vi "TDMS File Status.vi"(6 "Data Path":path=path "C:/Data", 8 "erriorIn":errorcluster, 9 "prefix":string, 11 "fileRefIn":refnum<k34>) -> (0 "error out":errorcluster, 3 "tdms file out":refnum<k34>)   [LabVIEW 2014]
uses:
  File Utilities.lvlib
panel:
  in  "nFile":bool
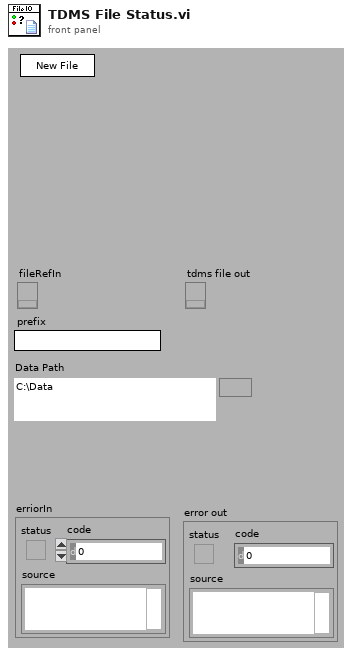
[diagram p1: front panel]
types:
  T1 = typedef "LVDateTimeRec.ctl" = cluster{"fractional second":dbl, "second":i32, "minute":i32, "hour":i32, "day of month":i32, "month":i32, "year":i32, "day of week":i32, "day of year":i32, "DST":i32}
  T2 = enum16{"open", "open or create", "create or replace", "create", "open (read-only)"}
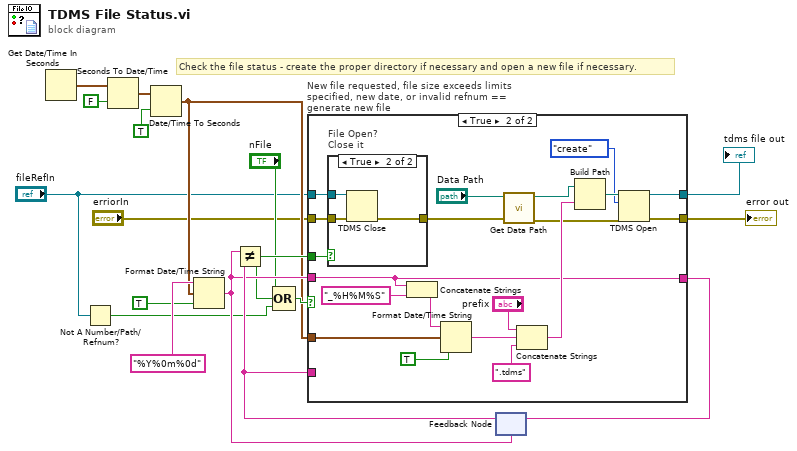
[diagram p0: block diagram]
diagram:
  # "Check the file status - create the proper directory if necessary and open a new file if necessary."
  n1 = Get Date/Time In Seconds() -> (seconds since 1Jan1904=w10:timestamp)
  n2 = Not A Number/Path/Refnum?(number/path/refnum="fileRefIn") -> (NaN/Path/Refnum?=w11:bool)
  n3 = Seconds To Date/Time(time stamp (now)=w10, to UTC (F)=FALSE) -> (date time rec=w7:T1)
  n4 = Date/Time To Seconds(1:TRUE ("is UTC (F)"), 2:w7) -> (0:w6:timestamp)
  n5 = Format Date/Time String(time format string (%c)="%Y%0m%0d", seconds (now)=w6, UTC format=TRUE) -> (date/time string=w15:string)
  n6 = feedback #1(w15) -> (w16:string)
  n7 = Not Equal?(x=w15, y=w16) -> (x != y?=w14:bool)
  n8 = Compound Arithmetic op=OR("nFile", w14, w11) -> (w13:bool)
  n9 = case "New file requested, file size exceeds limits specified, new date, or invalid refnum == generate new file" shown="True" w13 {
    tunnel: [w21 w33] -> w18
    tunnel: w15 -> [_ w33]
    tunnel: w14 -> [_ w41]
    tunnel: [w20 w24] -> w4
    tunnel: w16 -> [w21 _]
    tunnel: "erriorIn" -> [w20 w39]
    tunnel: w6 -> [_ w35]
    tunnel: [w19 w23] -> w1
    tunnel: "fileRefIn" -> [w19 w31]
    frame False {
    }
    frame True {
      n10 = case "File Open?\nClose it" shown="True" w41 {
        tunnel: [w42 w43] -> w29
        tunnel: w39 -> [w42 w45]
        tunnel: w31 -> [_ w44]
        frame False {
        }
        frame True {
          n11 = TDMS Close(8:w45, 11:w44) -> (0:w43:errorcluster)  [unwired: 1 out]
        }
      }
      n12 = Concatenate Strings(w33, "_%H%M%S" ("time format string (%c)")) -> (w37:string)
      n13 = Format Date/Time String(time format string (%c)=w37, seconds (now)=w35, UTC format=TRUE) -> (date/time string=w32:string)
      n14 = call "Get Data Path.vi"("error in"=w29, "Data Path In"="Data Path") -> ("error out"=w22:errorcluster, "Data Path Out"=w40:path)  [unwired: 8 in]
      n15 = Concatenate Strings("prefix", w32, ".tdms" ("string")) -> (w38:string)
      n16 = Build Path(base path=w40, name or relative path=w38) -> (appended path=w26:path)
      n17 = TDMS Open(8:w22, 10:T2."create" ("operation (0:open)"), 11:w26) -> (0:w24:errorcluster, 3:w23:refnum<k34>)  [unwired: 4 in]
    }
  }
  "error out" <- w4
  "tdms file out" <- w1
  n18 = feedback-in #1(w18) -> ()
